vi "(SubVI) Viscosity of glycerol soultion calculation_YCC_ver2.vi"(0 "Volumn of water":dbl, 2 "Volumn of glycerol":dbl, 5 "Temperature (C)":dbl) -> (7 "Density of mix (kg/m^3)":dbl, 8 "Viscosity of mix (Pa*s)":dbl)   [LabVIEW 2014]
panel:
  out "Mass% of water":dbl
  out "V% of water":dbl
  out "Viscosity of water (Ps*s)":dbl
  out "Total mass (kg)":dbl
  out "Viscosity of glycerol (Ps*s)":dbl
  out "Mass% of glycerol":dbl
  out "Mass of glycerol (kg)":dbl
  out "Mass of water (kg)":dbl
  out "Density of water (kg/m^3)":dbl
  out "Density of glycerol (kg/m^3)":dbl
  out "V% of glycerol":dbl
  out "Total Volumn":dbl
  # "cP"
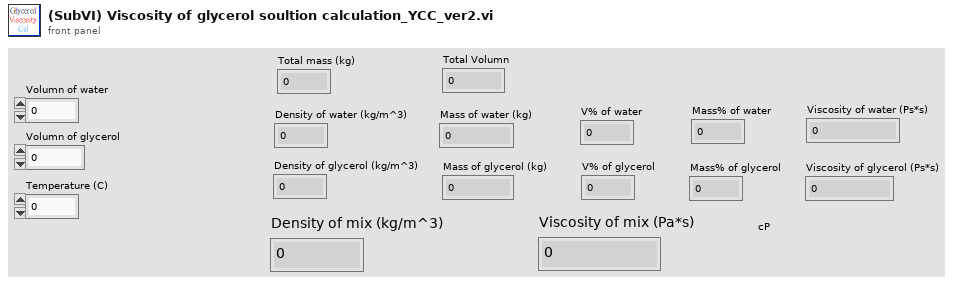
[diagram p1: front panel]
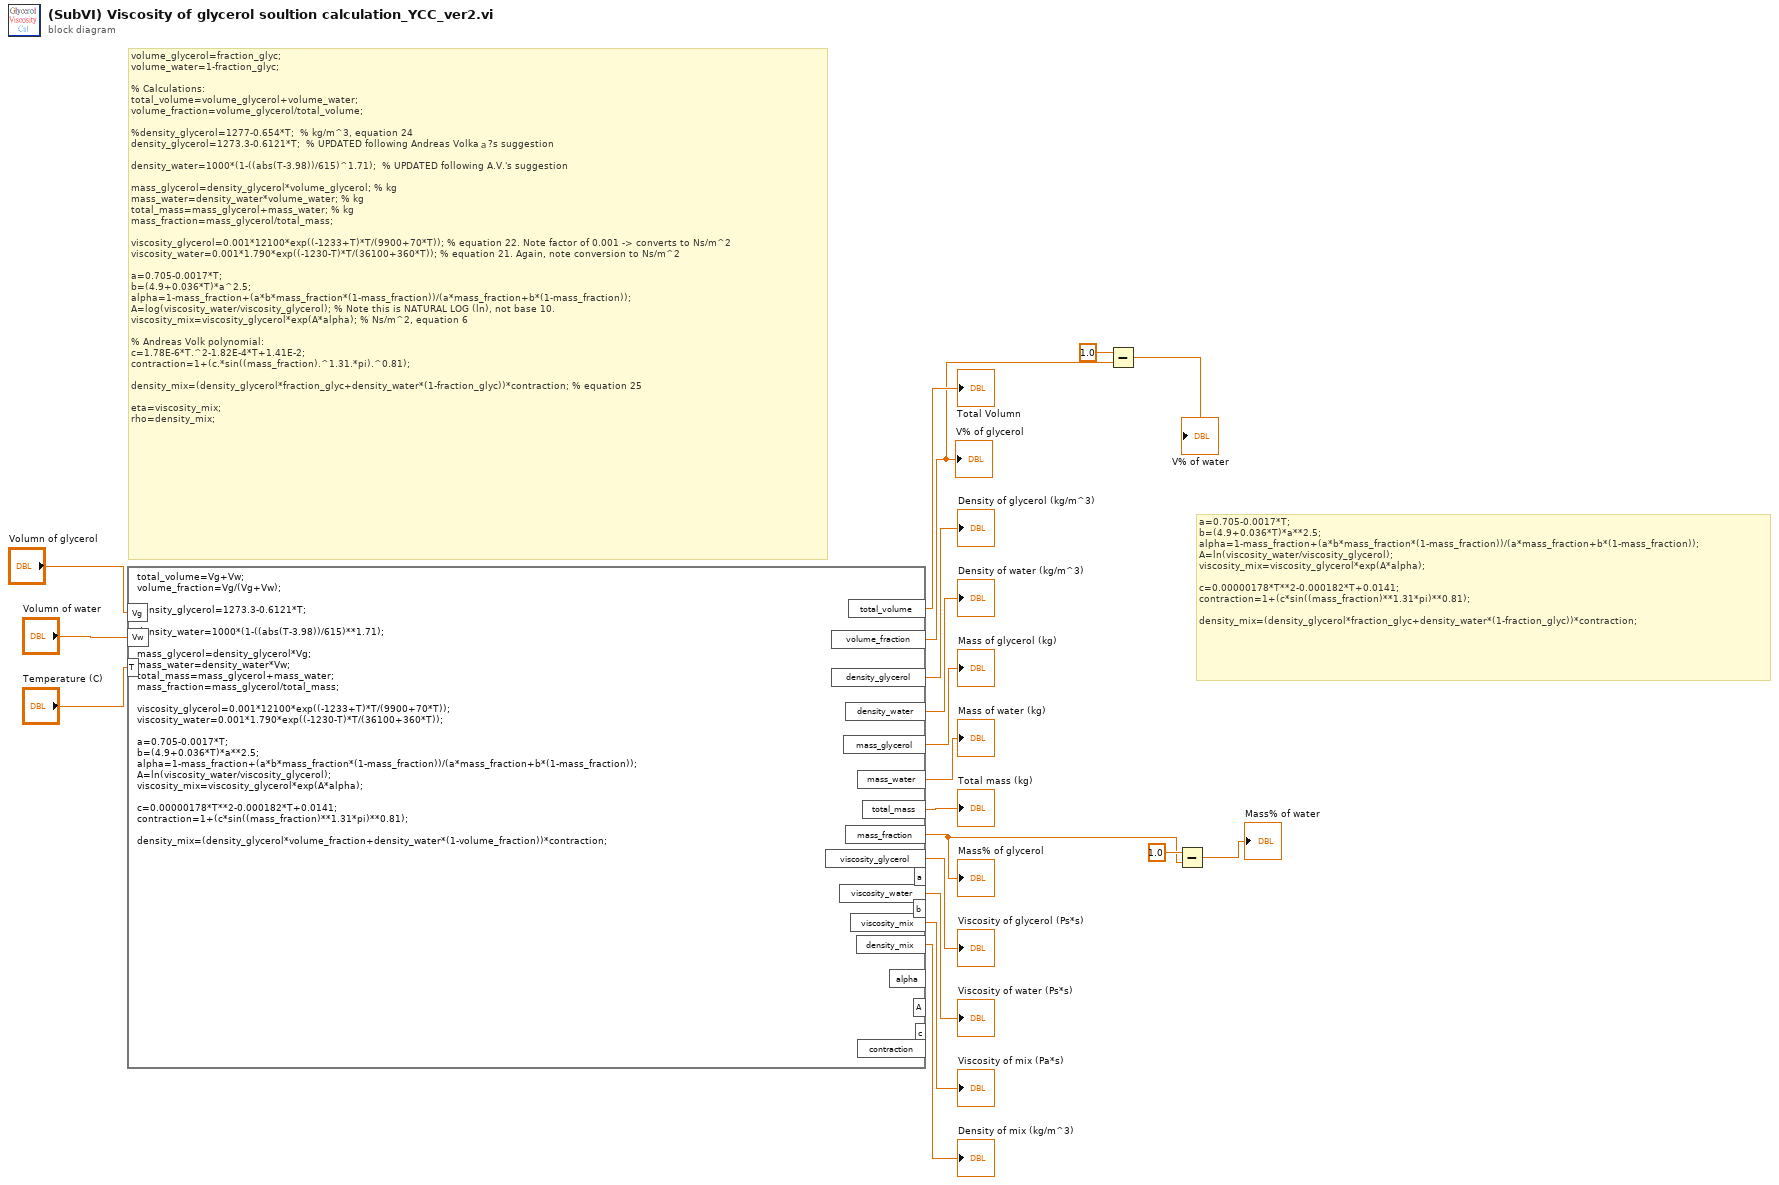
[diagram p0: block diagram]
diagram:
  # "a=0.705-0.0017*T;\nb=(4.9+0.036*T)*a**2.5;\nalpha=1-mass_fraction+(a*b*mass_fraction*(1-mass_fraction))/(a*mass_fraction+b*(1-mass_fraction));\nA=ln(viscosity_water/viscosity_glycerol); \nviscosity_mix=viscosity_glycerol*exp(A*alpha); \n\nc=0.00000178*T**2-0.000182*T+0.0141;\ncontraction=1+(c*sin((mass_fraction)**1.31*pi)**0.81);\n\ndensity_mix=(density_glycerol*fraction_glyc+density_water*(1-fraction_glyc))*contraction;"
  # "volume_glycerol=fraction_glyc;\nvolume_water=1-fraction_glyc;\n\n% Calculations:\ntotal_volume=volume_glycerol+volume_water;\nvolume_fraction=volume_glycerol/total_volume;\n\n%density_glycerol=1277-0.654*T;  % kg/m^3, equation 24\ndensity_glycerol=1273.3-0.6121*T;  % UPDATED following Andreas Volkaａ?s suggestion\n\ndensity_water=1000*(1-((abs(T-3.98))/615)^1.71);  % UPDATED following A.V.'s suggestion\n\nmass_glycerol=density_glycerol*volume_glycerol; % kg\nmass_water=density_water*volume_water; % kg\ntotal_mass=mass_glycerol+mass_water; % kg\nmass_fraction=mass_glycerol/total_mass;\n\nviscosity_glycerol=0.001*12100*exp((-1233+T)*T/(9900+70*T)); % equation 22. Note factor of 0.001 -> converts to Ns/m^2\nviscosity_water=0.001*1.790*exp((-1230-T)*T/(36100+360*T)); % equation 21. Again, note conversion to Ns/m^2\n\na=0.705-0.0017*T;\nb=(4.9+0.036*T)*a^2.5;\nalpha=1-mass_fraction+(a*b*mass_fraction*(1-mass_fraction))/(a*mass_fraction+b*(1-mass_fraction));\nA=log(viscosity_water/viscosity_glycerol); % Note this is NATURAL LOG (ln), not base 10.\nviscosity_mix=viscosity_glycerol*exp(A*alpha); % Ns/m^2, equation 6\n\n% Andreas Volk polynomial:\nc=1.78E-6*T.^2-1.82E-4*T+1.41E-2;\ncontraction=1+(c.*sin((mass_fraction).^1.31.*pi).^0.81);\n\ndensity_mix=(density_glycerol*fraction_glyc+density_water*(1-fraction_glyc))*contraction; % equation 25\n\neta=viscosity_mix;\nrho=density_mix;"
  n1 = formula code="total_volume=Vg+Vw;\nvolume_fraction=Vg/(Vg+Vw);\n\ndensity_glycerol=1273.3-0.6121*T;  \n\ndensity_water=1000*(1-((abs(T-3.98))/615)**1.71);  \n\nmass_glycerol=density_glycerol*Vg; \nmass_water=density_water*Vw; \ntotal_mass=mass_glycerol+mass_water; \nmass_fraction=mass_glycerol/total_mass;\n\nviscosity_glycerol=0.001*12100*exp((-1233+T)*T/(9900+70*T)); \nviscosity_water=0.001*1.790*exp((-1230-T)*T/(36100+360*T)); \n\na=0.705-0.0017*T;\nb=(4.9+0.036*T)*a**2.5;\nalpha=1-mass_fraction+(a*b*mass_fraction*(1-mass_fraction))/(a*mass_fraction+b*(1-mass_fraction));\nA=ln(viscosity_water/viscosity_glycerol); \nviscosity_mix=viscosity_glycerol*exp(A*alpha); \n\nc=0.00000178*T**2-0.000182*T+0.0141;\ncontraction=1+(c*sin((mass_fraction)**1.31*pi)**0.81);\n\ndensity_mix=(density_glycerol*volume_fraction+density_water*(1-volume_fraction))*contraction;"("Vg"="Volumn of glycerol", "Vw"="Volumn of water", "T"="Temperature (C)") -> ("total_volume"=→"Total Volumn":dbl, "volume_fraction"=w6:dbl, "density_glycerol"=→"Density of glycerol (kg/m^3)":dbl, "density_water"=→"Density of water (kg/m^3)":dbl, "mass_glycerol"=→"Mass of glycerol (kg)":dbl, "mass_water"=→"Mass of water (kg)":dbl, "total_mass"=→"Total mass (kg)":dbl, "mass_fraction"=w1:dbl, "viscosity_glycerol"=→"Viscosity of glycerol (Ps*s)":dbl, "viscosity_water"=→"Viscosity of water (Ps*s)":dbl, "viscosity_mix"=→"Viscosity of mix (Pa*s)":dbl, "density_mix"=→"Density of mix (kg/m^3)":dbl)  [unwired: 6 out]
  "V% of glycerol" <- w6
  "Mass% of glycerol" <- w1
  n2 = Subtract(x=1.0, y=w6) -> (x-y=→"V% of water":dbl)
  n3 = Subtract(x=1.0, y=w1) -> (x-y=→"Mass% of water":dbl)
